vi "Start Transaction.vi"(8 "error in":errorcluster, 11 "DB-MySQL in":refnum<class "DB-MySQL.lvclass">) -> (0 "error out":errorcluster, 3 "DB-MySQL out":refnum<class "DB-MySQL.lvclass">)   [LabVIEW 2014, in "hse-db.lvlib" / "DB-MySQL.lvclass"]
doc: "Start a transaction to get sure all following SQL commands get executed or none."
uses:
  DB-MySQL.lvclass
  DB-MySQL.lvclass/DB-MySQL.ctl
  DB-Engines/MySQLTcp/MySQL (TCP).lvlib
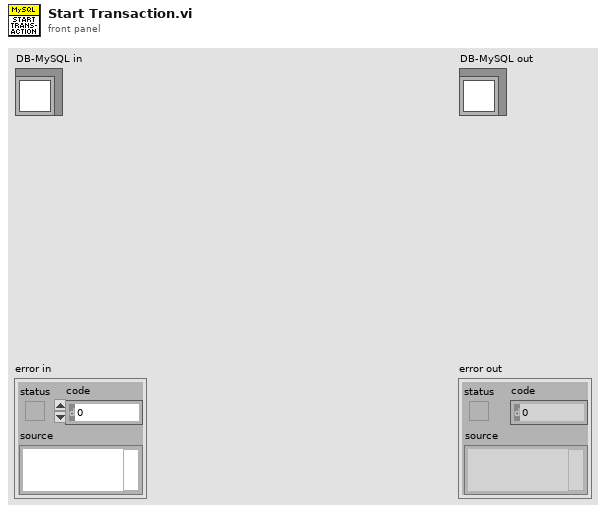
[diagram p1: front panel]
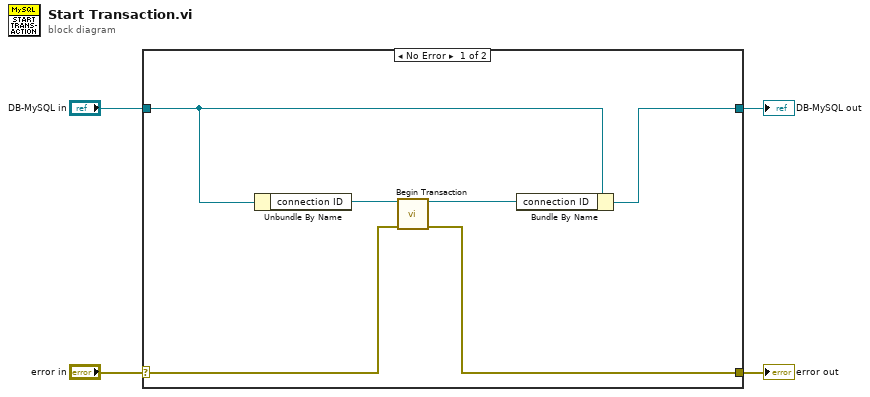
[diagram p0: block diagram]
diagram:
  n1 = case shown="No Error" "error in" {
    selector: "error in" -> [w10 w12]
    tunnel: [w9 w12] -> w3
    tunnel: [w6 w11] -> w1
    tunnel: "DB-MySQL in" -> [w7 w11]
    frame No Error {
      n2 = Unbundle By Name(w7) -> ("connection ID"=w8:refnum<k5>)
      n3 = call "Begin Transaction.vi"("connection ID in"=w8, "Error In"=w10) -> ("connection ID out"=w5:refnum<k5>, "Error Out"=w9:errorcluster)  [unwired: 12 in]
      n4 = Bundle By Name(cluster=w7, "connection ID"=w5) -> (w6:refnum<class "DB-MySQL.lvclass">)
    }
    frame Error {
    }
  }
  "error out" <- w3
  "DB-MySQL out" <- w1
